vi "DeadBand_(SubVI).vi"(9 "Axis In":i8, 10 "Deadband (10)":i8) -> (2 "Axis out":i8)   [LabVIEW 2012]
uses:
  <vilib>/NXT/Dual Mode Library/prims/inRangeAndCoerce/inRangeAndCoerce_int8.vi
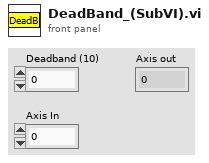
[diagram p1: front panel]
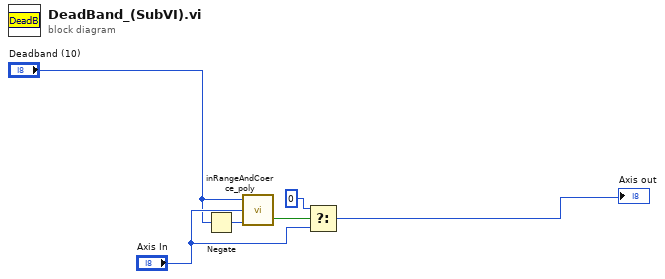
[diagram p0: block diagram]
diagram:
  n1 = Negate(x="Deadband (10)") -> (-x=w1:i8)
  n2 = call-poly <vilib>:"inRangeAndCoerce_poly.vi"("lower limit"=w1, "x"="Axis In", "upper limit"="Deadband (10)") -> ("In Range?"=w3:bool)  [unwired: 1 out]
  n3 = Select(t=i8 0, s=w3, f="Axis In") -> (s? t:f=→"Axis out":i8)
